vi "LS 340 Get Ramp.vi"(8 "error in (no error)":errorcluster, 10 "Output #":i32=1, 11 "VISA resource name":refnum<visa-resource-name>) -> (0 "error out":errorcluster, 1 "Ramp rate, K/min":dbl=1.0, 2 "Ramp on":bool, 3 "VISA Resource Name Out":refnum<visa-resource-name>)   [LabVIEW 2021]
uses:
  GPIB/VISA  Send Receive.vi
  Temperature Controller/Controls/Set Point Aproach.ctl
panel:
  out "data string out":string
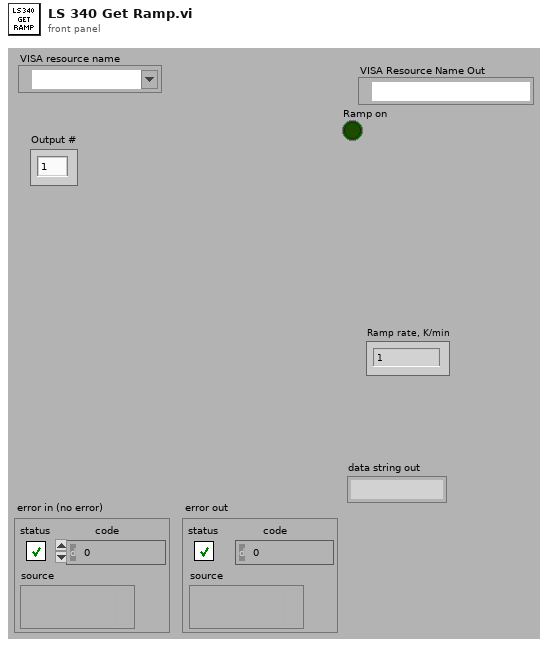
[diagram p1: front panel]
types:
  T1 = typedef "Set Point Aproach.ctl" = enum16{"Instant", "Ramp"}
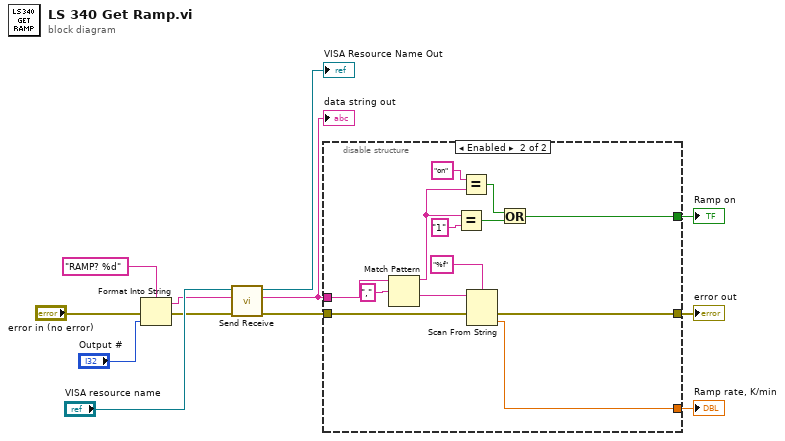
[diagram p0: block diagram]
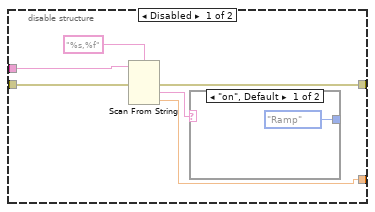
[diagram p2: hidden frame]
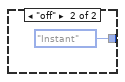
[diagram p3: hidden frame]
diagram:
  n1 = Format Into String(format string="RAMP? %d", error in="error in (no error)", "Output #") -> (resulting string=w2:string, error out=w5:errorcluster)  [unwired: 1 in]
  n2 = call-poly "Send Receive.vi"("error in (no error)"=w5, "data string in"=w2, "VISA Resource Name"="VISA resource name") -> ("error out"=w10:errorcluster, "data string out"=w7:string, "VISA Resource Name Out"=→"VISA Resource Name Out":refnum<visa-resource-name>)  [unwired: 6 in]
  "data string out" <- w7
  n3 = disable-structure shown="Enabled" {
    disable-tunnel: w10 -> [w19 w31]
    disable-tunnel: [w18 w30] -> w9
    disable-tunnel: [w15 w28] -> w6
    disable-tunnel: w7 -> [w14 w34]
    disable-tunnel: [_ w22] -> w1
    frame Disabled {
      n4 = Scan From String(format string="%s,%f", input string=w14, error in=w19) -> (error out=w18:errorcluster, output 1=w17:string, output 2=w15:dbl)  [unwired: 3 in, 2 out]
      n5 = case shown="\"on\", Default" w17 {
        tunnel: [Set_Point_Aproach."Ramp" ("Approach") Set_Point_Aproach."Instant" ("Approach")] -> w16
        frame "on", Default {
        }
        frame "off" {
        }
      }
    }
    frame Enabled {
      n6 = Match Pattern(string=w34, regular expression=",") -> (before substring=w25:string, after substring=w29:string)  [unwired: 1 in, 2 out]
      n7 = Equal?(x=w25, y="1" ("x")) -> (x = y?=w26:bool)
      n8 = Equal?(x="on", y=w25) -> (x = y?=w23:bool)
      n9 = Scan From String(format string="%f", input string=w29, error in=w31) -> (error out=w30:errorcluster, output 1=w28:dbl)  [unwired: 2 in, 2 out]
      n10 = Or(x=w23, y=w26) -> (x .or. y?=w22:bool)
    }
  }
  "error out" <- w9
  "Ramp rate, K/min" <- w6
  "Ramp on" <- w1
